vi "Test Variant2Str.vi"() -> ()   [LabVIEW 2020]
panel:
  out "Control Name":string
  out "variant output":variant
  in  "Variant":variant
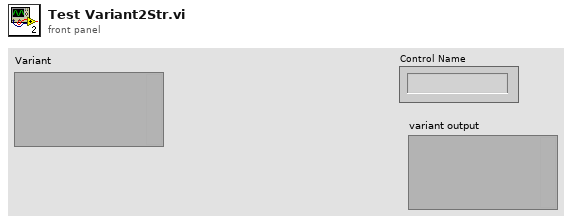
[diagram p1: front panel]
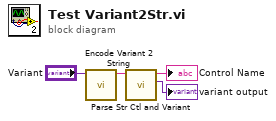
[diagram p0: block diagram]
diagram:
  n1 = call "Encode Variant 2 String.vi"("Variant"="Variant") -> ("String Output"=w4:string)  [unwired: 9 in, 1 out]
  n2 = call "Parse Str Ctl and Variant.vi"("String Input"=w4) -> ("variant output"=→"variant output":variant, "Control Name"=→"Control Name":string)  [unwired: 8 in, 1 out]
